vi "simx Display Dialog.vi"(0 "clientID":i32, 1 "titleText":string, 2 "mainText":string, 3 "dialogType":i32, 4 "initialText":string, 5 "titleColors":sgl, 6 "dialogColors":sgl, 7 "error in (no error)":errorcluster, 8 "dialogHandle":i32, 9 "uiHandle":i32, 10 "operationMode":i32) -> (18 "dialogHandle out":i32, 19 "uiHandle out":i32, 20 "function return":i32, 27 "error out":errorcluster)   [LabVIEW 2019, in "PXL_V-REP.lvlib"]
doc: "EXTAPI_DLLEXPORT simxInt simxDisplayDialog(simxInt clientID,const simxChar* titleText,const simxChar* mainText,simxInt dialogType,const simxChar* initialText,const simxFloat* titleColors,const simxFloat* dialogColors,simxInt* dialogHandle,simxInt* uiHandle,simxInt operationMode);"
uses:
  PXL_V-REP.lvlib
  <userlib>/V-REP/remoteApi.dll
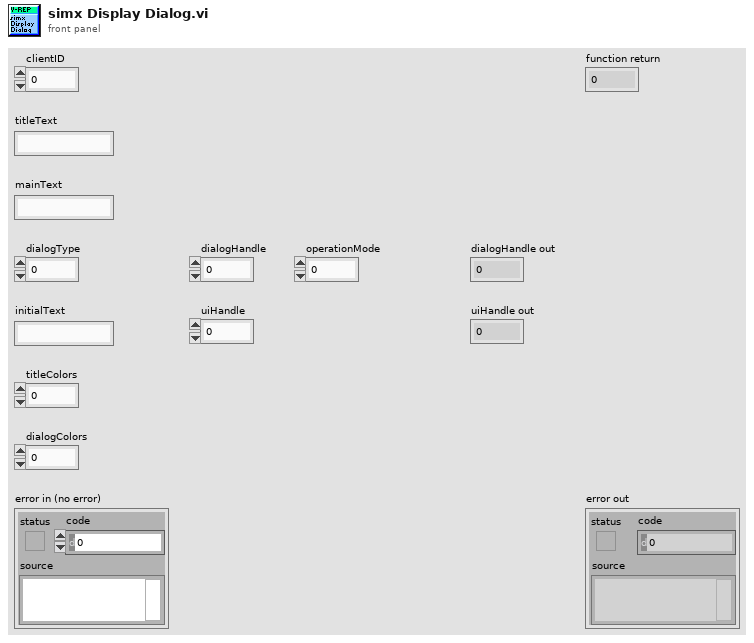
[diagram p1: front panel]
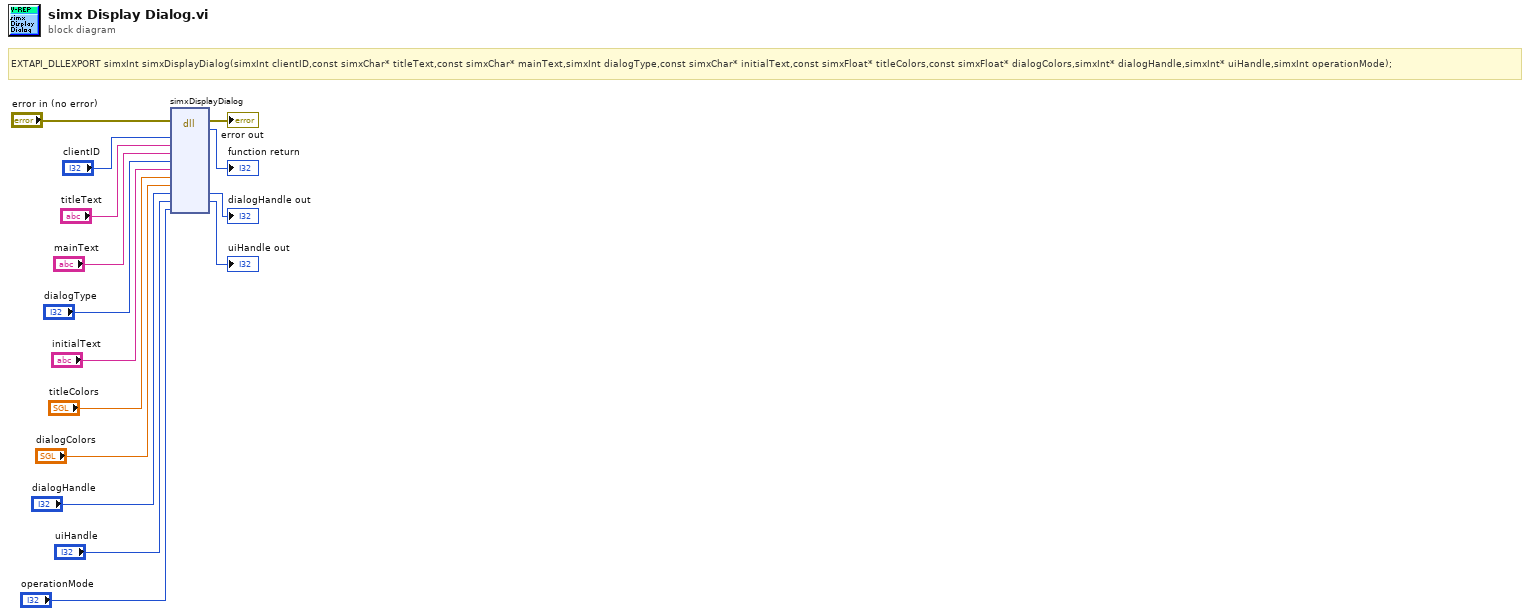
[diagram p0: block diagram]
diagram:
  # "EXTAPI_DLLEXPORT simxInt simxDisplayDialog(simxInt clientID,const simxChar* titleText,const simxChar* mainText,simxInt dialogType,const simxChar* initialText,const simxFloat* titleColors,const simxFloat* dialogColors,simxInt* dialogHandle,simxInt* uiHandle,simxInt operationMode);"
  n1 = dll-call lib="C:/Program Files (x86)/National Instruments/LabVIEW 2019/user.lib/V-REP/remoteApi.*" fn="simxDisplayDialog"(error in="error in (no error)", "clientID"="clientID", "titleText"="titleText", "mainText"="mainText", "dialogType"="dialogType", "initialText"="initialText", "titleColors"="titleColors", "dialogColors"="dialogColors", "dialogHandle"="dialogHandle", "uiHandle"="uiHandle", "operationMode"="operationMode") -> (error out=→"error out":errorcluster, →"function return":i32, "dialogHandle"=→"dialogHandle out":i32, "uiHandle"=→"uiHandle out":i32)  [unwired: 10 in, 1 out]
